vi "Fill RT Alarm Log Table.vi"(11 "Alarm Log":i16[](array[numeric])) -> (3 "appended array":string[](array[string]))   [LabVIEW 2018]
panel:
  out "# record":string
  out "description":string
  out "alarm code":string
  out "alarm type":string
  out "time":string
  out "date":string
  out "alarm code":i16
  out "alarm type":i16
  out "sec ms":i16
  out "hr min":i16
  out "moth day":i16
  out "year":i16
  out "record":i16
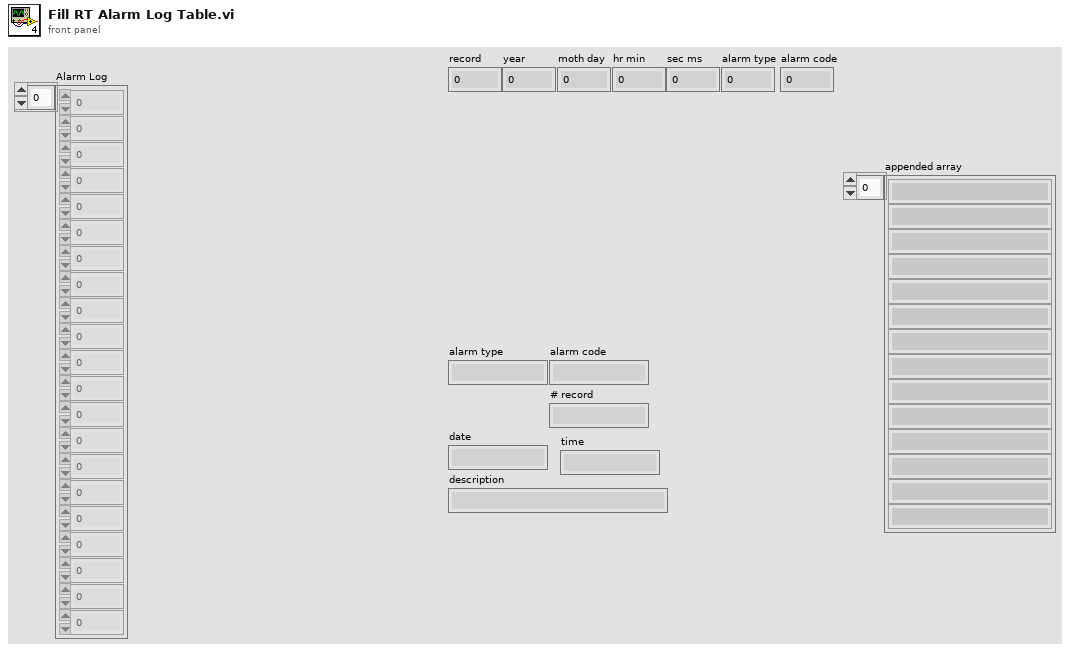
[diagram p1: front panel]
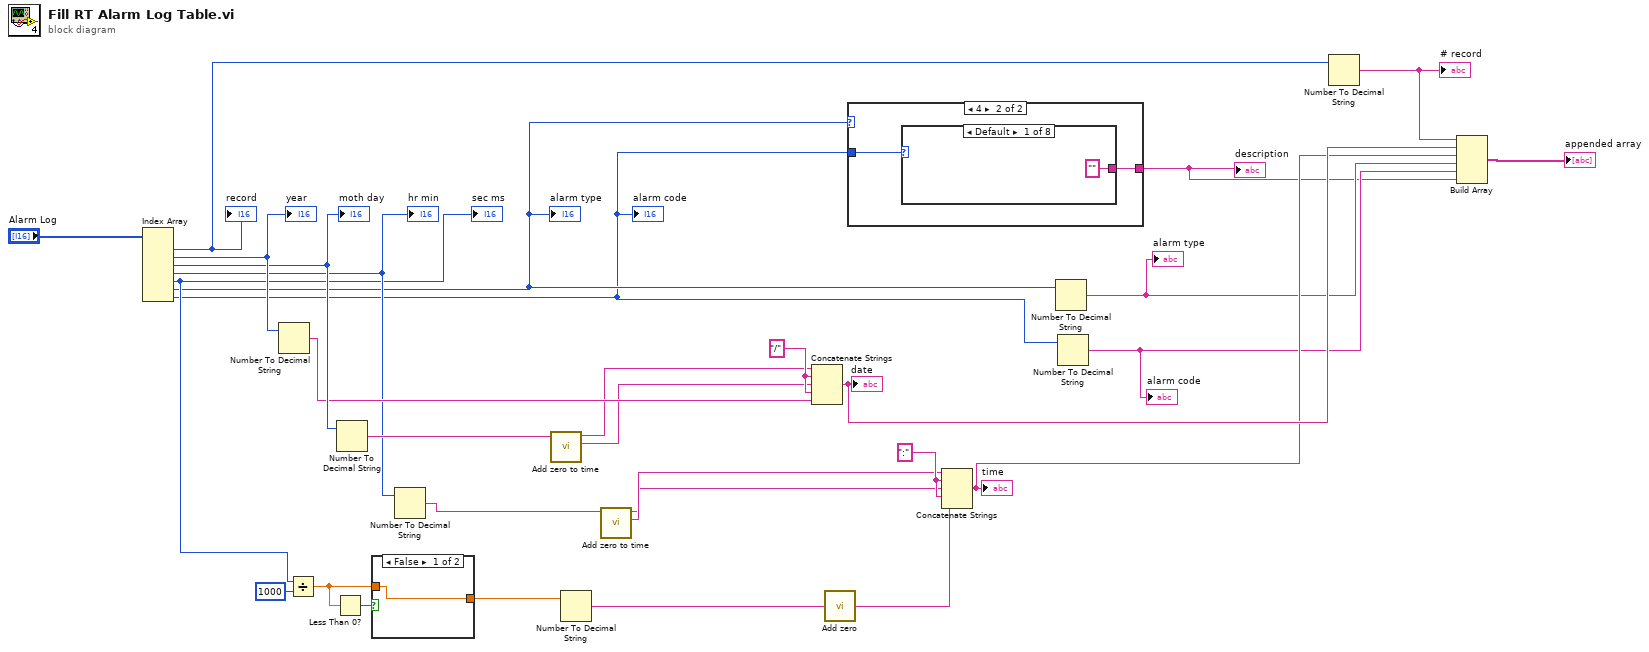
[diagram p0: block diagram]
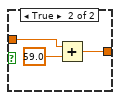
[diagram p2: hidden frame]
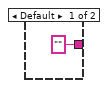
[diagram p3: hidden frame]
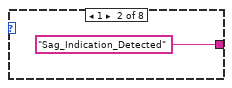
[diagram p4: hidden frame]
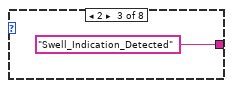
[diagram p5: hidden frame]
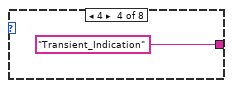
[diagram p6: hidden frame]
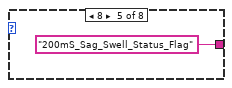
[diagram p7: hidden frame]
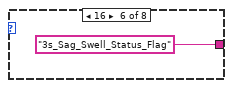
[diagram p8: hidden frame]
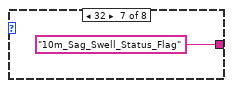
[diagram p9: hidden frame]
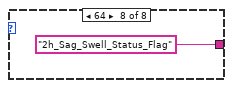
[diagram p10: hidden frame]
diagram:
  w19 = ":"
  w26 = "/"
  n1 = Index Array(array="Alarm Log") -> (element #1=w16:i16, element #2=w29:i16, element #3=w28:i16, element #4=w22:i16, element #5=w20:i16, element #6=w18:i16, element #7=w17:i16)  [unwired: 7 in]
  "record" <- w16
  "year" <- w29
  "moth day" <- w28
  "hr min" <- w22
  "sec ms" <- w20
  "alarm type" <- w18
  "alarm code" <- w17
  n2 = Number To Decimal String(number=w29) -> (decimal integer string=w25:string)  [unwired: 1 in]
  n3 = Divide(x=w20, y=i16 1000) -> (x/y=w4:dbl)
  n4 = Less Than 0?(x=w4) -> (x < 0?=w3:bool)
  n5 = Number To Decimal String(number=w28) -> (decimal integer string=w27:string)  [unwired: 1 in]
  n6 = case shown="False" w3 {
    tunnel: w4 -> [w31 w34]
    tunnel: [w31 w32] -> w2
    frame False {
    }
    frame True {
      n7 = Add(x=w34, y=59.0) -> (x+y=w32:dbl)
    }
  }
  n8 = Number To Decimal String(number=w22) -> (decimal integer string=w7:string)  [unwired: 1 in]
  n9 = call "Add zero to time.vi"("in"=w27) -> ("value 2"=w24:string, "value 1"=w23:string)  [unwired: 9 in]
  n10 = Number To Decimal String(number=w2) -> (decimal integer string=w21:string)  [unwired: 1 in]
  n11 = call "Add zero to time.vi"("in"=w7) -> ("value 2"=w6:string, "value 1"=w5:string)  [unwired: 9 in]
  n12 = Concatenate Strings(w23, w26, w24, w26, w25) -> (w14:string)
  "date" <- w14
  n13 = call "Add zero.vi"("in"=w21) -> ("out"=w1:string)
  n14 = case shown="4" w18 {
    tunnel: w17 -> [_ w37]
    tunnel: ["" w36] -> w10
    frame Default {
    }
    frame 4 {
      n15 = case shown="Default" w37 {
        tunnel: ["" "Sag_Indication_Detected" "Swell_Indication_Detected" "Transient_Indication" "200mS_Sag_Swell_Status_Flag" "3s_Sag_Swell_Status_Flag" "10m_Sag_Swell_Status_Flag" "2h_Sag_Swell_Status_Flag"] -> w36
        frame Default {
        }
        frame 1 {
        }
        frame 2 {
        }
        frame 4 {
        }
        frame 8 {
        }
        frame 16 {
        }
        frame 32 {
        }
        frame 64 {
        }
      }
    }
  }
  "description" <- w10
  n16 = Concatenate Strings(w6, w19, w5, w19, w1) -> (w13:string)
  "time" <- w13
  n17 = Number To Decimal String(number=w18) -> (decimal integer string=w12:string)  [unwired: 1 in]
  "alarm type" <- w12
  n18 = Number To Decimal String(number=w17) -> (decimal integer string=w11:string)  [unwired: 1 in]
  "alarm code" <- w11
  n19 = Number To Decimal String(number=w16) -> (decimal integer string=w15:string)  [unwired: 1 in]
  "# record" <- w15
  n20 = Build Array(w15, w14, w13, w12, w11, w10) -> (→"appended array":string[])
